vi "Handle Filter Automation.vi"(11 "Controller in":refnum<class "Controller.lvclass">) -> ()   [LabVIEW 2018, in "Controller.lvlib" / "Controller.lvclass"]
doc: "This Controller method uses a DVR containing a switch object to determine whether the filter should be automatically switched. The state of the DVR (whether to cycle, what the period of the cycle is, what the length of the filter is, etc) is maintained in the messaging loop. In this VI, the current state is checked, and if time has elapsed and the switch is set to cycle, a message is sent to the main message loop to change the state."
uses:
  Controller.lvclass
  C:/Program Files (x86)/National Instruments/LabVIEW 2018/vi.lib/ActorFramework/Actor/Actor.lvclass
  C:/Users/Labview/Documents/exscalabar_server/SuperActor/SuperActor.lvclass
  <vilib>/Platform/TimedLoop/XDataNode/timing_clust.ctl
  <vilib>/Platform/TimedLoop/XDataNode/nitl_modes.ctl
  <vilib>/Platform/TimedLoop/XDataNode/wakeup.ctl
  <vilib>/ActorFramework/Actor/Actor.lvclass/Actor.ctl
  <vilib>/ActorFramework/Message Enqueuer/Message Enqueuer.lvclass/Message Enqueuer.ctl
  Controller.lvclass/Controller.ctl
  SuperActor/SuperActor.lvclass/SuperActor.ctl
  Messages/Change Filter State/Change Filter State.lvclass
  C:/Users/Labview/Documents/exscalabar_server/Controller/Messages/Update Switch State MSG/Update Switch MSG.lvclass
  C:/Program Files (x86)/National Instruments/LabVIEW 2018/vi.lib/ActorFramework/Message/Message.lvclass
  Messages/Update Switch State MSG/Update Switch MSG.lvclass/Update Switch MSG.ctl
  Controls/eMap.ctl
  <vilib>/ActorFramework/Message Enqueuer/Message Enqueuer.lvclass
  Instr Actor/Messages/Change Speaker State/Change Speaker Switch MSG.lvclass
  Messages/Update Switch State MSG/Write SwitchState.vi
  SuperActor/Read CVT Session.vi
  Accessors/Read Enqueuer Map.vi
  <vilib>/ActorFramework/Message Enqueuer/Init from Existing Queue.vi
  <vilib>/ActorFramework/Message Priority Queue/Priority Enqueue.vi
  <userlib>/_Session Fwk/Session - Root.lvclass
  <vilib>/Platform/TimedLoop/XDataNode/XDataNode.xnode
  reusable/Switch/Switch.lvclass
  <vilib>/Platform/TimedLoop/XDataNode/XDNodeRunTimeDep.lvlib
  <vilib>/ActorFramework/Actor/Actor.lvclass
  reusable/Session APIs/CVT/CVT.lvclass
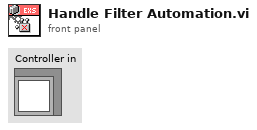
[diagram p1: front panel]
types:
  T1 = typedef "Session - Root.lvclass/Session Handle.ctl" = refnum<data-value>
  T2 = typedef "XDNodeRunTimeDep.lvlib/timing_clust.ctl" = cluster{"Expected End [f-1]":u64, "Actual End [f-1]":u64, "Finished Late? [f-1]":bool, "Expected End [i-1]":u64, "Actual End [i-1]":u64, "Finished Late? [i-1]":bool, "Expected Start [i]":u64, "Actual Start [i]":u64, "Expected Start [f]":u64, "Actual Start [f]":u64, "Source Name":string, "Structure Name":string, "Period":i64, "Deadline":i64, "Offset":i64, "Start":i64, "Priority":i32, "Timeout":i32, "Mode":T3, "Wakeup Reason":T4, "Error":errorcluster, "Source Type":string, "Secondary Source Type":string, "Global End Time":u64, "Global Start Time":u64, "Frame Duration":u64, "Iteration Duration":u64, "Assigned CPU":i32, "I/O Scan Engine Mode":u32}
  T3 = typedef "XDNodeRunTimeDep.lvlib/nitl_modes.ctl" = enum32{"No Change", "Process missed periods, maintain original phase", "Discard missed periods, maintain original phase", "Process missed periods, ignore original phase", "Discard missed periods, ignore original phase"}
  T4 = typedef "XDNodeRunTimeDep.lvlib/wakeup.ctl" = enum32{"Normal", "Aborted", "Asynchronous wakeup", "Timing source error", "Timed loop error", "Timeout"}
  T5 = typedef "Controller.lvlib/Controller.lvclass/eMap.ctl" = cluster{"Enqueuer":refnum<class "Message Enqueuer.lvclass">, "Active":bool}
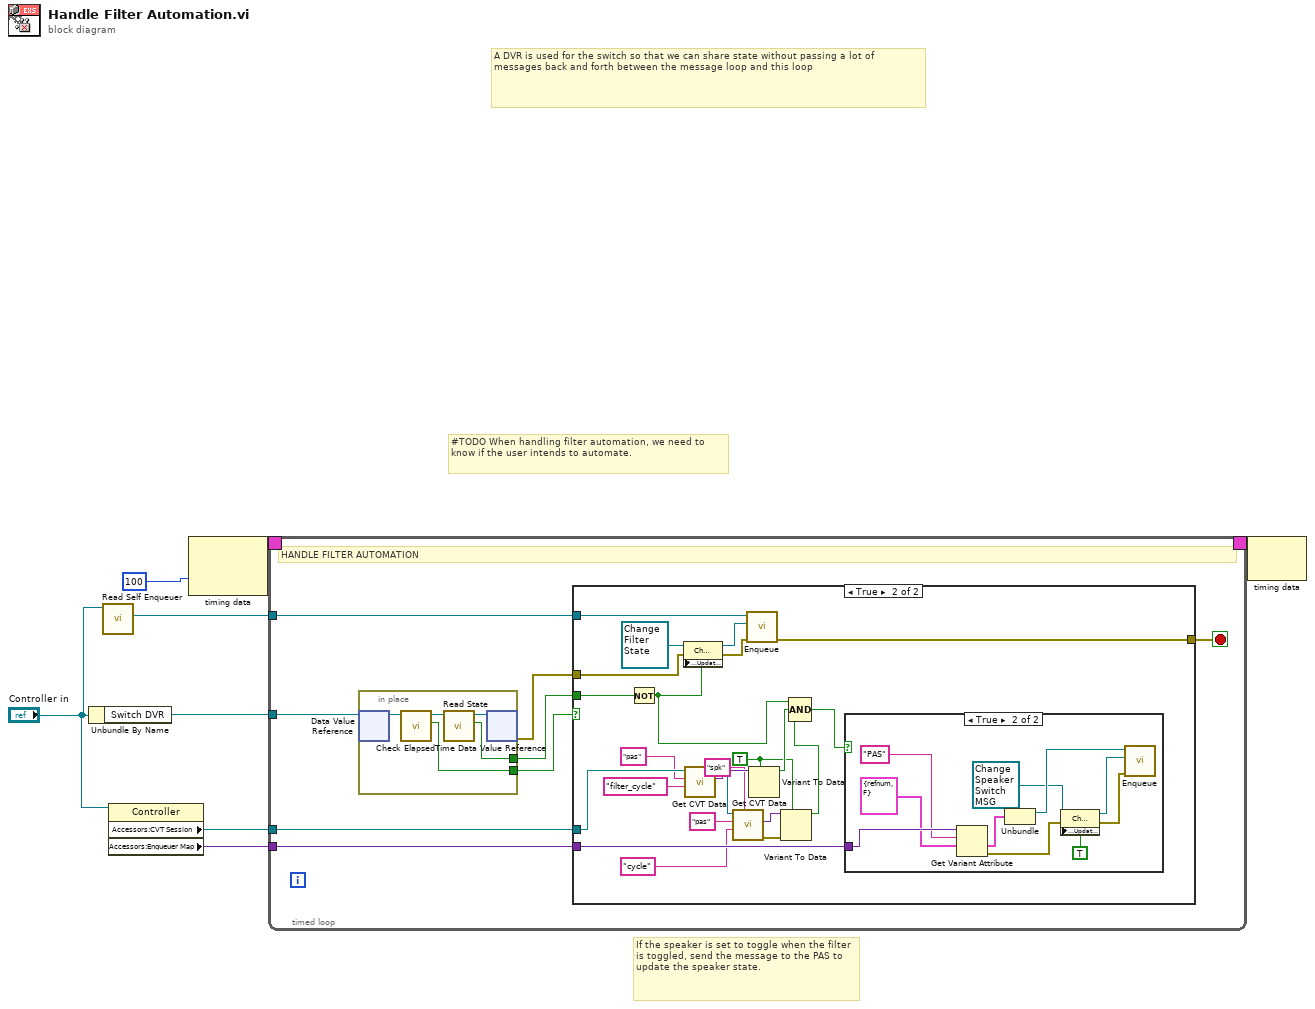
[diagram p0: block diagram]
diagram:
  # "If the speaker is set to toggle when the filter is toggled, send the message to the PAS to update the speaker state."
  # "A DVR is used for the switch so that we can share state without passing a lot of messages back and forth between the message loop and this loop"
  # "#TODO When handling filter automation, we need to know if the user intends to automate."
  n1 = Unbundle By Name("Controller in") -> ("Switch DVR"=w5:refnum<data-value>)
  n2 = call <vilib>:"Read Self Enqueuer.vi"("Actor"="Controller in") -> ("Self Enqueuer"=w4:refnum<class "Message Enqueuer.lvclass">)  [unwired: 10 in]
  n3 = property class="Controller"(reference="Controller in") -> ("Accessors:CVT Session"=w2:T1, "Accessors:Enqueuer Map"=w1:variant)  [unwired: 1 in, 2 out]
  n4 = node-c288(i64 100 ("Period")) -> (w8:T2)  [unwired: 1 in]
  n5 = timed-loop {
    timing: w8 -> [_]
    timing-out: [_] -> w7
    tunnel: w5 -> [w16]
    tunnel: w4 -> [w13]
    tunnel: w2 -> [w10]
    tunnel: w1 -> [w9]
    stop <- w11 stop-if-true
    # "HANDLE FILTER AUTOMATION"
    n6 = in-place {
      in-place-border: [w54] -> w15
      in-place-border: [w51] -> w14
      n7 = in-place-dvr #1(w16) -> (w55:refnum<class "Switch.lvclass">)  [unwired: 1 out]
      n8 = call-dynamic "Check ElapsedTime.vi"("Switch in"=w55) -> ("Cycle Switch?"=w54:bool, "Switch out"=w53:refnum<class "Switch.lvclass">)  [unwired: 7 in, 2 out]
      n9 = call-dynamic "Read State.vi"("Switch in"=w53) -> ("State"=w51:bool, "Switch out"=w52:refnum<class "Switch.lvclass">)  [unwired: 8 in, 1 out]
      n10 = in-place-dvr #1(w52) -> (w12:errorcluster)  [unwired: 1 out]
    }
    n11 = case shown="True" w15 {
      tunnel: w14 -> [_ w40]
      tunnel: w13 -> [_ w37]
      tunnel: w12 -> [w17 w36]
      tunnel: [w17 w34] -> w11
      tunnel: w10 -> [_ w33]
      tunnel: w9 -> [_ w29]
      frame False {
      }
      frame True {
        w20 = TRUE
        n12 = Not(x=w40) -> (.not. x?=w27:bool)
        n13 = property class="Change Filter State MSG"(reference=refnum<class "Change Filter State.lvclass"> refnum ("Controller.lvlib:Change Filter State.lvclass"), error in=w36, "Accessors:UpdateSw"=w27) -> (reference out=w38:refnum<class "Change Filter State.lvclass">, error out=w35:errorcluster)
        n14 = call "Get CVT Data.vi"("Variable"="filter_cycle", "Group"="pas" ("Subgroup"), "CVT Session In"=w33) -> ("Data Out"=w30:variant, "CVT Session Out"=w25:T1)  [unwired: 5 in, 2 out]
        n15 = call "Get CVT Data.vi"("Subgroup"="spk", "Variable"="cycle" ("Group"), "Group"="pas", "CVT Session In"=w25) -> ("error out"=w22:errorcluster, "Data Out"=w21:variant)  [unwired: 4 in, 2 out]
        n16 = call <vilib>:"Enqueue.vi"("error in (no error)"=w35, "Message"=w38, "Message Enqueuer in"=w37) -> ("error out"=w34:errorcluster)  [unwired: 7 in, 1 out]
        n17 = Variant To Data(type=w20, Variant=w30) -> (data=w28:bool)  [unwired: 1 in, 1 out]
        n18 = Variant To Data(error in=w22, type=w20, Variant=w21) -> (data=w19:bool)  [unwired: 1 out]
        n19 = Compound Arithmetic op=AND(w27, w28, w19) -> (w26:bool)
        n20 = case shown="True" w26 {
          tunnel: w29 -> [_ w50]
          frame False {
          }
          frame True {
            n21 = Get Variant Attribute(Variant=w50, name="PAS", default value (empty Variant)=T5 {"Enqueuer"=refnum, "Active"=FALSE} ("eMap")) -> (value=w47:T5, error out=w42:errorcluster)  [unwired: 1 in, 2 out]
            n22 = Unbundle(w47) -> ("Enqueuer"=w46:refnum<class "Message Enqueuer.lvclass">)  [unwired: 1 out]
            n23 = property class="Change Speaker MSG"(reference=refnum<class "Change Speaker Switch MSG.lvclass"> refnum ("ePAS Library.lvlib:Change Speaker MSG"), error in=w42, "Accessors:UpdateSw"=TRUE ("UpdateSw")) -> (reference out=w43:refnum<class "Change Speaker Switch MSG.lvclass">, error out=w41:errorcluster)
            n24 = call <vilib>:"Enqueue.vi"("error in (no error)"=w41, "Message"=w43, "Message Enqueuer in"=w46) -> ()  [unwired: 7 in, 2 out]
          }
        }
      }
    }
  }
  n25 = node-c288(w7) -> ()  [unwired: 1 out]
